vi "SimpleExampleOOP(MM).vi"() -> ()   [LabVIEW 2013]
uses:
  StellarNetSpecAcquisitionClass/StellarNetSpecAcquisition.lvclass
  StellarNetSpectrometerClass/StellarNetSpectrometer.lvclass
panel:
  out "Spectrum":sgl[](graph)
  out "OK":bool
  in  "stop":bool
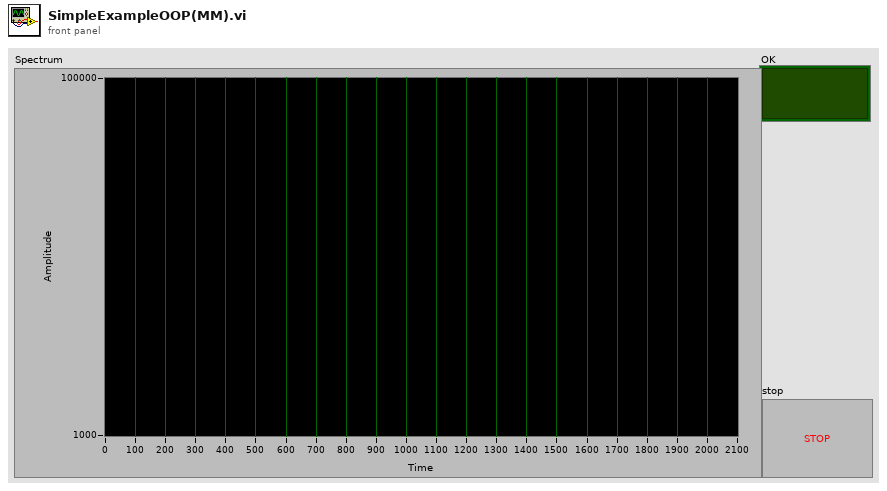
[diagram p1: front panel]
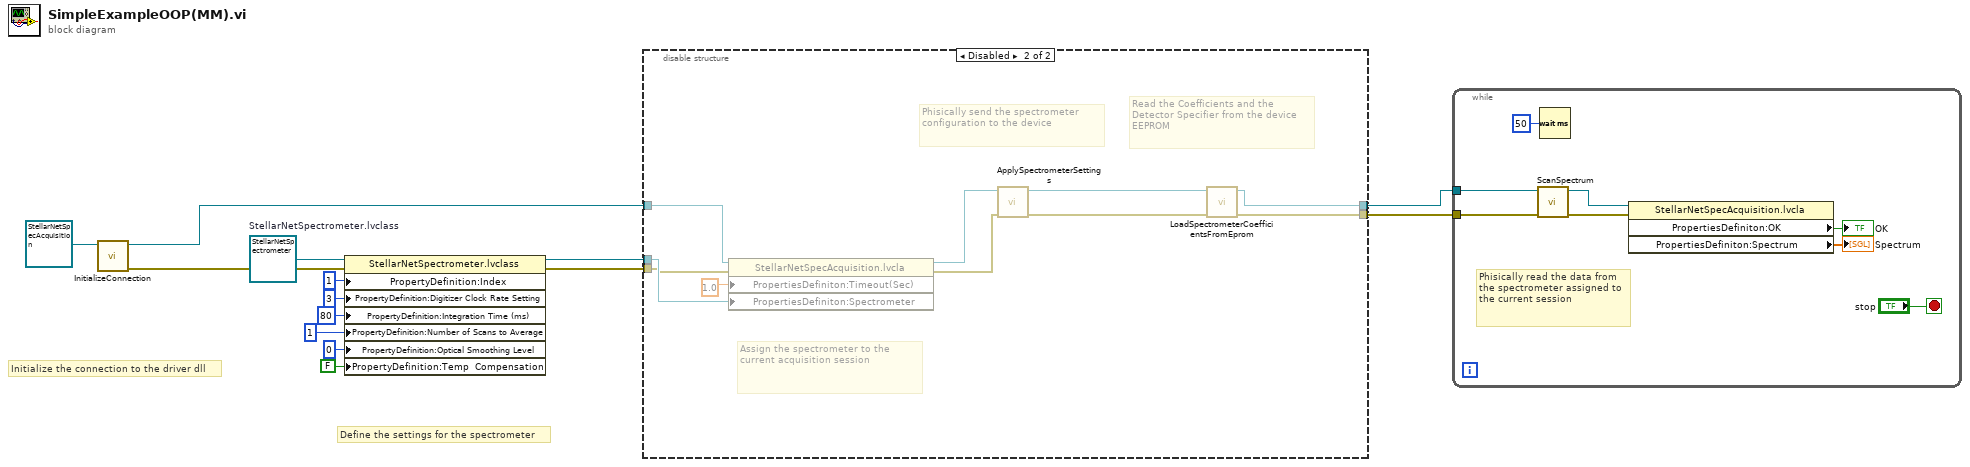
[diagram p0: block diagram]
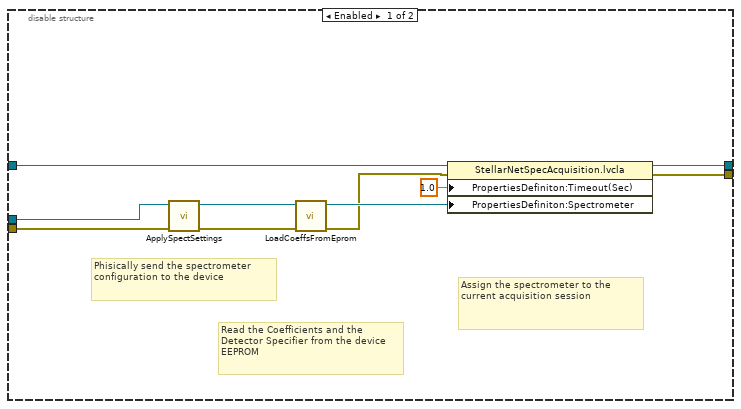
[diagram p2: hidden frame]
diagram:
  w14 = refnum<class "StellarNetSpectrometer.lvclass"> refnum  # StellarNetSpectrometer.lvclass
  # "Initialize the connection to the driver dll"
  # "Define the settings for the spectrometer"
  n1 = call-dynamic "InitializeConnection.vi"("StellarNetSpecAcquisition in"=refnum<class "StellarNetSpecAcquisition.lvclass"> refnum ("StellarNetSpecAcquisition.lvclass")) -> ("error out"=w1:errorcluster, "StellarNetSpecAcquisition out"=w2:refnum<class "StellarNetSpecAcquisition.lvclass">)  [unwired: 9 in]
  n2 = property class="StellarNetSpectrometer.lvclass"(reference=w14, error in=w1, "PropertyDefinition:Index"=u32 1 ("Index"), "PropertyDefinition:Digitizer Clock Rate Setting"=3 ("Digitizer Clock Rate Setting"), "PropertyDefinition:Integration Time (ms)"=80 ("Integration Time (ms)"), "PropertyDefinition:Number of Scans to Average"=1 ("Number of Scans to Average"), "PropertyDefinition:Optical Smoothing Level"=0 ("Optical Smoothing Level"), "PropertyDefinition:Temp  Compensation "=FALSE ("Temp  Compensation")) -> (reference out=w5:refnum<class "StellarNetSpectrometer.lvclass">, error out=w4:errorcluster)
  n3 = disable-structure shown="Disabled" {
    disable-tunnel: [w24 w26] -> w7
    disable-tunnel: [w23 w25] -> w6
    disable-tunnel: w5 -> [w22 w28]
    disable-tunnel: w4 -> [w21 w27]
    disable-tunnel: w2 -> [w20 w29]
    frame Enabled {
      # "Assign the spectrometer to the current acquisition session"
      # "Read the Coefficients and the Detector Specifier from the device EEPROM"
      # "Phisically send the spectrometer configuration to the device"
      n4 = call-dynamic "ApplySpectSettings.vi"("error in"=w21, "StellarNetSpectrometer in"=w22) -> ("error out"=w19:errorcluster, "StellarNetSpectrometer out"=w18:refnum<class "StellarNetSpectrometer.lvclass">)  [unwired: 8 in]
      n5 = call-dynamic "LoadCoeffsFromEprom.vi"("error in"=w19, "StellarNetSpectrometer in"=w18) -> ("error out"=w16:errorcluster, "StellarNetSpectrometer out"=w17:refnum<class "StellarNetSpectrometer.lvclass">)  [unwired: 8 in]
      n6 = property class="StellarNetSpecAcquisition.lvcla"(reference=w20, error in=w16, "PropertiesDefiniton:Timeout(Sec)"=1.0 ("Timeout(Sec)"), "PropertiesDefiniton:Spectrometer"=w17) -> (reference out=w23:refnum<class "StellarNetSpecAcquisition.lvclass">, error out=w24:errorcluster)
    }
    frame Disabled {
      # "Assign the spectrometer to the current acquisition session"
      # "Read the Coefficients and the Detector Specifier from the device EEPROM"
      # "Phisically send the spectrometer configuration to the device"
      n7 = property class="StellarNetSpecAcquisition.lvcla"(reference=w29, error in=w27, "PropertiesDefiniton:Timeout(Sec)"=1.0 ("Timeout(Sec)"), "PropertiesDefiniton:Spectrometer"=w28) -> (reference out=w31:refnum<class "StellarNetSpecAcquisition.lvclass">, error out=w32:errorcluster)
      n8 = call-dynamic "ApplySpectrometerSettings.vi"("error in (no error)"=w32, "StellarNetSpecAcquisition in"=w31) -> ("error out"=w34:errorcluster, "StellarNetSpecAcquisition out"=w33:refnum<class "StellarNetSpecAcquisition.lvclass">)  [unwired: 8 in]
      n9 = call-dynamic "LoadSpectrometerCoefficientsFromEprom.vi"("error in (no error)"=w34, "StellarNetSpecAcquisition in"=w33) -> ("error out"=w26:errorcluster, "StellarNetSpecAcquisition out"=w25:refnum<class "StellarNetSpecAcquisition.lvclass">)  [unwired: 8 in]
    }
  }
  n10 = while {
    tunnel: w7 -> [w42]
    tunnel: w6 -> [w41]
    stop <- "stop" stop-if-true
    # "Phisically read the data from the spectrometer assigned to the current session"
    n11 = call-dynamic "ScanSpectrum.vi"("error in"=w42, "StellarNetSpecAcquisition in"=w41) -> ("error out"=w39:errorcluster, "StellarNetSpecAcquisition out"=w40:refnum<class "StellarNetSpecAcquisition.lvclass">)  [unwired: 8 in]
    n12 = Wait (ms)(milliseconds to wait=u32 50) -> ()  [unwired: 1 out]
    n13 = property class="StellarNetSpecAcquisition.lvcla"(reference=w40, error in=w39) -> ("PropertiesDefiniton:OK"=→"OK":bool, "PropertiesDefiniton:Spectrum"=→"Spectrum":sgl[])  [unwired: 2 out]
  }
